vi "Case not matched.vi"(0 "Case Name not Matched":string) -> ()   [LabVIEW 2020]
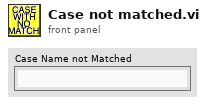
[diagram p1: front panel]
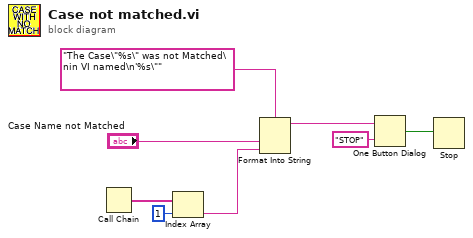
[diagram p0: block diagram]
diagram:
  n1 = Call Chain() -> (call chain=w3:string[])
  n2 = Index Array(array=w3, index=1) -> (element=w1:string)
  n3 = Format Into String(format string="The Case\"%s\" was not Matched\nin VI named\n'%s\"" ("Format String"), "Case Name not Matched", w1) -> (resulting string=w5:string)  [unwired: 2 in, 1 out]
  n4 = One Button Dialog(message=w5, button name ("OK")="STOP") -> (true=w7:bool)
  n5 = Stop(stop? (T)=w7) -> ()
